vi "Save Load Notes.vi"(0 "Load Notes":string[](array[string]), 5 "Load#":i32, 7 "Log?":bool, 9 "Time":timestamp[](array[timestamp]), 11 "error in (no error)":errorcluster) -> (15 "error out":errorcluster)   [LabVIEW 2015]
uses:
  <vilib>/addons/_office/excel.llb/Excel Easy Table (str).vi
  <vilib>/Utility/NIReport.llb/NI_report.lvclass
  <vilib>/addons/_office/NI_ReportGenerationToolkit.lvlib
  <vilib>/Utility/NIReport.llb/Excel/NI_Excel.lvclass
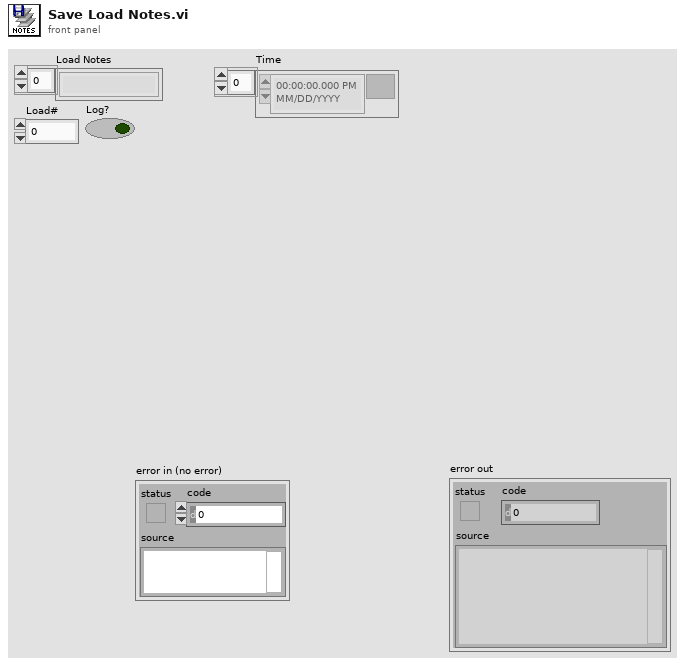
[diagram p1: front panel]
types:
  T1 = enum16{"maximized", "minimized", "normal", "no change"}
  T2 = enum16{"Standard Report", "HTML", "Word", "Excel"}
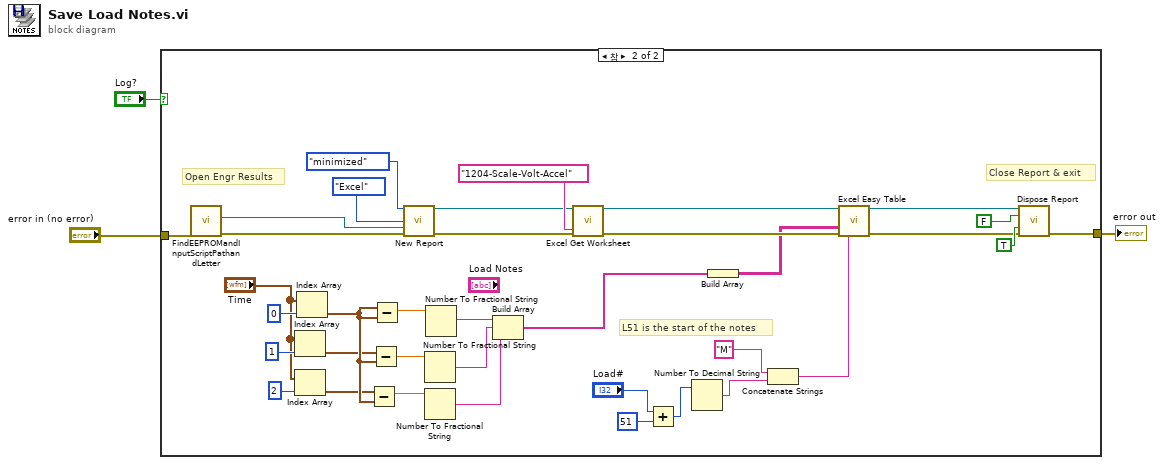
[diagram p0: block diagram]
diagram:
  n1 = case shown="참" "Log?" {
    tunnel: "error in (no error)" -> [w4 w32]
    tunnel: [w4 w28] -> w2
    frame False {
    }
    frame True {
      # "L51 is the start of the notes"
      # "Close Report & exit"
      # "Open Engr Results"
      n2 = call "FindEEPROMandInputScriptPathandLetter.vi"("Error In"=w32) -> ("Error Out"=w31:errorcluster, "Engr Result Path"=w40:path)  [unwired: 6 in, 1 out]
      n3 = Index Array(array="Time", index=1) -> (element=w13:timestamp)
      n4 = Index Array(array="Time", index=2) -> (element=w12:timestamp)
      n5 = Index Array(array="Time", index=0) -> (element=w14:timestamp)
      n6 = Subtract(x=w12, y=w14) -> (x-y=w9:dbl)
      n7 = Subtract(x=w13, y=w14) -> (x-y=w10:dbl)
      n8 = Subtract(x=w14, y=w14) -> (x-y=w11:dbl)
      n9 = call <vilib>:"New Report.vi"("window state (normal)"=T1."minimized", "report type"=T2."Excel", "template (empty)"=w40, "error in (no error)"=w31) -> ("report out"=w34:refnum<class "NI_report.lvclass">, "error out"=w33:errorcluster)  [unwired: 10 in]
      n10 = Number To Fractional String(number=w10) -> (F-format string=w7:string)  [unwired: 3 in]
      n11 = Number To Fractional String(number=w9) -> (F-format string=w6:string)  [unwired: 3 in]
      n12 = Number To Fractional String(number=w11) -> (F-format string=w8:string)  [unwired: 3 in]
      n13 = Build Array(w8, w7, w6) -> (w5:string[])
      n14 = call <vilib>:"Excel Get Worksheet.vi"("report in"=w34, "error in (no error)"=w33, "name (\"\")"="1204-Scale-Volt-Accel" ("name (\"\")")) -> ("report out"=w30:refnum<class "NI_report.lvclass">, "error out"=w29:errorcluster)  [unwired: 11 in]
      n15 = Add(x="Load#", y=51) -> (x+y=w22:i32)
      n16 = Number To Decimal String(number=w22) -> (decimal integer string=w21:string)  [unwired: 1 in]
      n17 = Build Array(w5) -> (w25:string[][])
      n18 = Concatenate Strings("M" ("name (\"\")"), w21) -> (w19:string)
      n19 = call-poly <vilib>:"Excel Easy Table.vi"("report in"=w30, "text data"=w25, "error in (no error)"=w29, "name (\"\")"=w19) -> ("report out"=w27:refnum<class "NI_report.lvclass">, "error out"=w26:errorcluster)  [unwired: 7 in, 3 out]
      n20 = call-dynamic "Dispose Report.vi"("report in"=w27, "wait until printing completed? (T)"=FALSE, "save changes? (F)"=TRUE, "error in (no error)"=w26) -> ("error out"=w28:errorcluster)  [unwired: 11 in]
    }
  }
  "error out" <- w2
